vi "Delete Active Graphic.vi"(8 "error in (no error)":errorcluster, 11 "Canvas in":refnum<class "Canvas.lvclass">) -> (0 "error out":errorcluster, 3 "Canvas out":refnum<class "Canvas.lvclass">)   [LabVIEW 2015, in "Canvas.lvclass"]
uses:
  Canvas.lvclass
  Canvas.lvclass/Canvas.ctl
  Graphic/Graphic.lvclass/Graphic.ctl
  Graphic/Graphic.lvclass
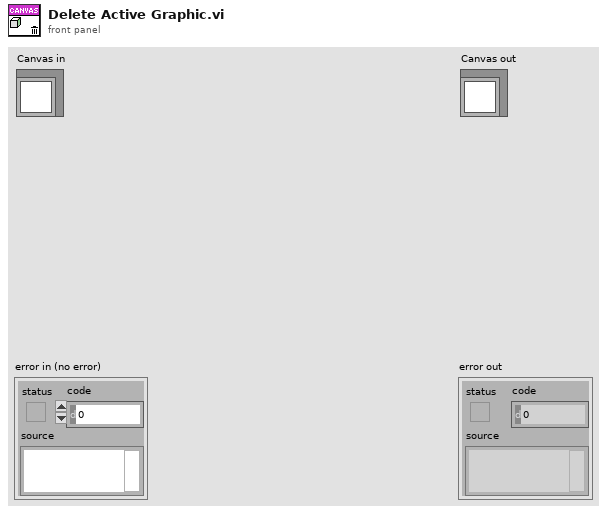
[diagram p1: front panel]
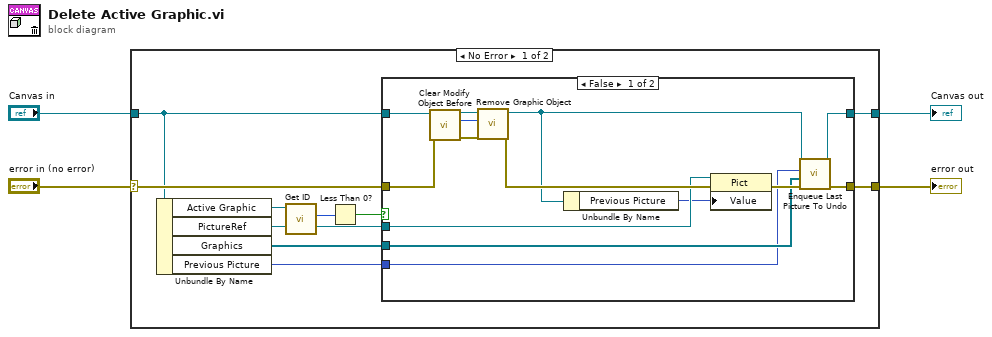
[diagram p0: block diagram]
diagram:
  n1 = case shown="No Error" "error in (no error)" {
    selector: "error in (no error)" -> [w14 w32]
    tunnel: [w12 w32] -> w3
    tunnel: [w13 w31] -> w1
    tunnel: "Canvas in" -> [w11 w31]
    frame No Error {
      n2 = Unbundle By Name(w11) -> ("Active Graphic"=w10:refnum<class "Graphic.lvclass">, "PictureRef"=w7:refnum<vi>, "Graphics"=w6:refnum<class "Graphic.lvclass">[], "Previous Picture"=w5:picture)
      n3 = call "Get ID.vi"("Graphic in"=w10) -> ("ID"=w9:i32)  [unwired: 8 in, 2 out]
      n4 = Less Than 0?(x=w9) -> (x < 0?=w8:bool)
      n5 = case shown="False" w8 {
        tunnel: w14 -> [w26 w29]
        tunnel: [w24 w30] -> w13
        tunnel: [w22 w29] -> w12
        tunnel: w11 -> [w21 w30]
        tunnel: w7 -> [w18 _]
        tunnel: w6 -> [w16 _]
        tunnel: w5 -> [w15 _]
        frame False {
          n6 = call "Clear Modify Object Before.vi"("error in (no error)"=w26, "Canvas in"=w21) -> ("error out"=w25:errorcluster, "ID"=w27:i32, "Canvas out"=w28:refnum<class "Canvas.lvclass">)  [unwired: 7 in]
          n7 = call "Remove Graphic Object.vi"("error in (no error)"=w25, "ID"=w27, "Canvas in"=w28) -> ("error out"=w23:errorcluster, "Canvas out"=w20:refnum<class "Canvas.lvclass">)  [unwired: 7 in]
          n8 = Unbundle By Name(w20) -> ("Previous Picture"=w17:picture)
          n9 = property class="Pict"(reference=w18, error in=w23, "Value"=w17) -> (error out=w19:errorcluster)  [unwired: 1 out]
          n10 = call "Enqueue Last Picture To Undo.vi"("error in (no error)"=w19, "Graphics"=w16, "Last Picture"=w15, "Canvas in"=w20) -> ("error out"=w22:errorcluster, "Canvas out"=w24:refnum<class "Canvas.lvclass">)  [unwired: 6 in]
        }
        frame True {
        }
      }
    }
    frame Error {
    }
  }
  "error out" <- w3
  "Canvas out" <- w1
